vi "AddDatapoint_real.vi"(3 "error in (no error)":errorcluster, 4 "Sensor info":string[][](array[string]), 5 "Sensor Type":string, 6 "connection reference in":T1) -> (0 "error out":errorcluster, 1 "Temperature":dbl, 2 "connection reference out":T1)   [LabVIEW 2023]
uses:
  <vilib>/addons/database/Connection.llb/Conn ObjectReference.ctl
  <vilib>/addons/database/Connection.llb/Conn Execute.vi
  <vilib>/addons/database/Recordset.llb/Rec Destroy - Connection.vi
  <vilib>/addons/database/NI_Database_API.lvlib
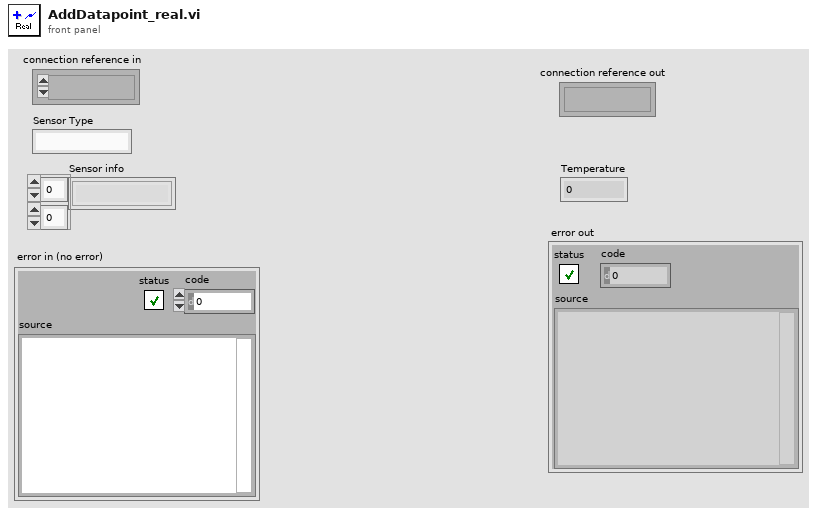
[diagram p1: front panel]
types:
  T1 = typedef "NI_Database_API.lvlib/Conn ObjectReference.ctl" = refnum<k1>
  T2 = typedef "NI_Database_API.lvlib/Rec ObjectReference.ctl" = refnum<k1>
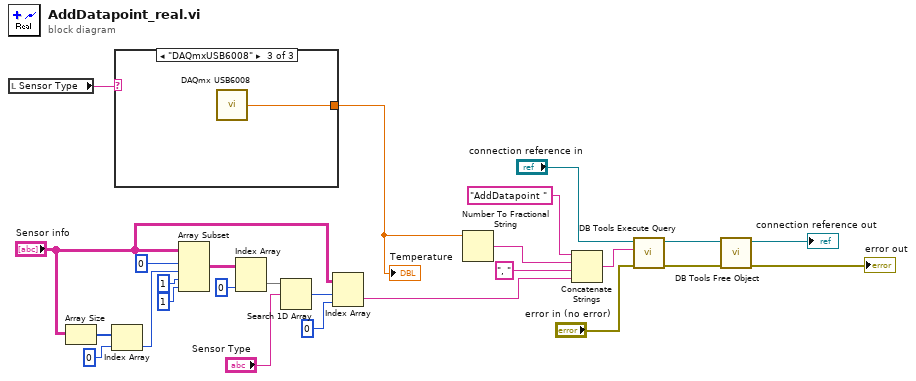
[diagram p0: block diagram]
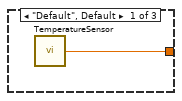
[diagram p2: hidden frame]
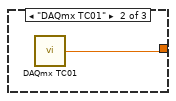
[diagram p3: hidden frame]
diagram:
  n1 = local read "Sensor Type"() -> (w1:string)
  n2 = Array Size(array="Sensor info") -> (size(s)=w12:i32[])
  n3 = Index Array(array=w12, index=0) -> (element=w3:i32)
  n4 = case shown="\"DAQmxUSB6008\"" w1 {
    tunnel: [w27 w28 w29] -> w16
    frame "Default", Default {
      n5 = call "TemperatureSensor.vi"() -> ("Temperature"=w27:dbl)  [unwired: 1 in]
    }
    frame "DAQmx TC01" {
      n6 = call "DAQmx TC01.vi"() -> ("Temperature data"=w28:dbl)  [unwired: 1 in]
    }
    frame "DAQmxUSB6008" {
      n7 = call "DAQmx USB6008.vi"() -> ("Temperature data"=w29:dbl)  [unwired: 1 in]
    }
  }
  "Temperature" <- w16
  n8 = Array Subset(array="Sensor info", index (row)=0 ("index"), length (row)=w3, index (col)=1 ("index"), length (col)=1 ("length")) -> (w4:string[][])
  n9 = Index Array(array=w4, index (col)=0 ("dimension size")) -> (element=w5:string[])  [unwired: 1 in]
  n10 = Search 1D Array(1D array=w5, element="Sensor Type") -> (index of element=w6:i32)  [unwired: 1 in]
  n11 = Index Array(array="Sensor info", index (row)=w6, index (col)=0 ("index")) -> (element=w2:string)
  n12 = Number To Fractional String(number=w16) -> (F-format string=w24:string)  [unwired: 3 in]
  n13 = Concatenate Strings("AddDatapoint " ("string"), w24, ", " ("string"), w2) -> (w23:string)
  n14 = call-poly <vilib>:"DB Tools Execute Query.vi"("error in (no error)"="error in (no error)", "SQL query"=w23, "connection reference"="connection reference in") -> ("error out"=w26:errorcluster, "recordset reference"=w25:T2)  [unwired: 5 in]
  n15 = call-poly <vilib>:"DB Tools Free Object.vi"("error in (no error)"=w26, "recordset reference"=w25) -> ("error out"=→"error out":errorcluster, "connection reference"=→"connection reference out":T1)  [unwired: 8 in]
